vi "ELVIS-RIO Customized FPGA.vi"() -> ()   [LabVIEW 2016]
doc: "This VI contains the NI myRIO FPGA shipping personality. This VI compiles and runs on the NI myRIO FPGA target. You can modify this VI to suit your application needs. National Instruments recommends that you only add new FPGA code to this VI and do not modify the existing code. This VI might not work correctly with the myRIO VIs if you modify the existing code."
uses:
  <vilib>/Platform/TimedLoop/XDataNode/timing_clust.ctl
  <vilib>/Platform/TimedLoop/XDataNode/nitl_modes.ctl
  <vilib>/Platform/TimedLoop/XDataNode/wakeup.ctl
  <vilib>/rvi/eio/common/nirviEmuTemplateMethod_errors.vi
  <vilib>/rvi/interface/RandomDataEmulation/niFpgaRandomDataHandleErrors.vi
  <vilib>/rvi/Emulation/niFpgaCriticalErrorInLSC.vi
  <vilib>/rvi/Emulation/niFpgaGetClockAttributes.vi
  <vilib>/rvi/Emulation/niFpgaEmulationReportErrorSimple.vi
  <vilib>/rvi/Emulation/niFpgaSctlEmulationGetInTimedLoop.vi
  <vilib>/rvi/Emulation/niFpgaProcessEmulError.vi
  <vilib>/Platform/TimedLoop/XDataNode/XDataNode.xnode
  <vilib>/eio/EIONode/EIONode.xnode
  <vilib>/rvi/DataTransferAndStorage/Container/XNode/niFpgaContainer.xnode
  <vilib>/rvi/interface/RandomDataEmulation/nirviRandomDataFpgaReadWriteTemplate.vi
  <vilib>/Platform/TimedLoop/XDataNode/XDNodeRunTimeDep.lvlib
panel:
  in  "Encoder 1 Reset Value":i32
  in  "Encoder 0 Reset Value":i32
  in  "Calibrated":bool
  out "Encoder 0 Counter":i32
  out "Encoder 1 Counter":i32
  in  "Encoder 1 Reset":bool
  in  "Encoder 0 Reset":bool
  out "24V Error":bool
  in  "Camera Power":bool
  in  "LED3 Yellow":bool
  in  "LED2 Yellow":bool
  in  "LED1 Yellow":bool
  out "FIFO Receive Time Out":bool
  out "Framing Error":bool
  in  "Clear Framing Error":bool
  in  "UART Clock Divisor":u16
  in  "PWM0 Enable":bool
  out "Stall Warning 0":bool
  out "Stall Error 0":bool
  out "Encoder 0 Raw":fxp<+,2,2> format="%02b"
  out "Encoder 1 Raw":fxp<+,2,2> format="%02b"
  in  "PWM1 Enable":bool
  in  "LED1 Red":bool
  in  "LED2 Green":bool
  in  "LED2 Red":bool
  in  "LED1 Green":bool
  in  "LED3 Red":bool
  in  "LED3 Green":bool
  out "Stall Warning 1":bool
  out "Stall Error 1":bool
  out "myRIO Button":u8 format="%08b"
  in  "myRIO LED3:0":u8 format="%04b"
  in  "PWM.1A":u16
  in  "PWM.1B":u16
  in  "PWM.0A":u16
  in  "PWM.0B":u16
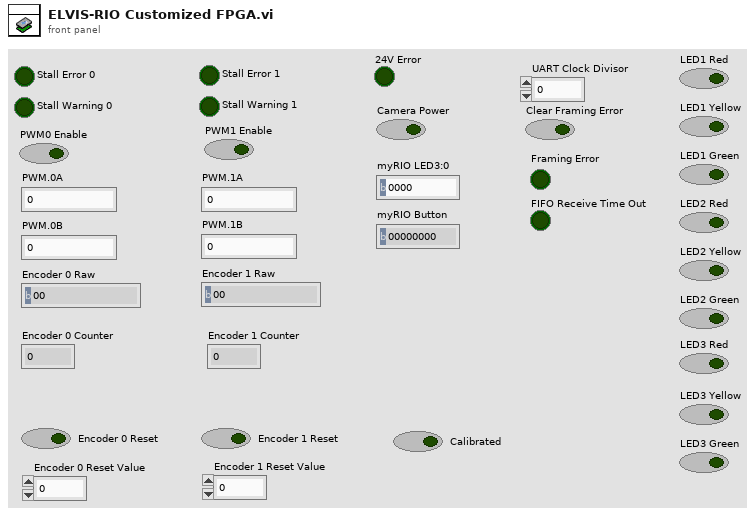
[diagram p1: front panel]
types:
  T1 = enum16{"Idle", "Testing Start", "Finish Start", "Data", "FIFO Data", "Testing Stop"}
  T2 = enum16{"Idle", "Send Bit", "Wait for Baud Period"}
  T3 = typedef "XDNodeRunTimeDep.lvlib/timing_clust.ctl" = cluster{"Expected End [f-1]":u64, "Actual End [f-1]":u64, "Finished Late? [f-1]":bool, "Expected End [i-1]":u64, "Actual End [i-1]":u64, "Finished Late? [i-1]":bool, "Expected Start [i]":u64, "Actual Start [i]":u64, "Expected Start [f]":u64, "Actual Start [f]":u64, "Source Name":string, "Structure Name":string, "Period":i64, "Deadline":i64, "Offset":i64, "Start":i64, "Priority":i32, "Timeout":i32, "Mode":T4, "Wakeup Reason":T5, "Error":errorcluster, "Source Type":string, "Secondary Source Type":string, "Global End Time":u64, "Global Start Time":u64, "Frame Duration":u64, "Iteration Duration":u64, "Assigned CPU":i32, "I/O Scan Engine Mode":u32}
  T4 = typedef "XDNodeRunTimeDep.lvlib/nitl_modes.ctl" = enum32{"No Change", "Process missed periods, maintain original phase", "Discard missed periods, maintain original phase", "Process missed periods, ignore original phase", "Discard missed periods, ignore original phase"}
  T5 = typedef "XDNodeRunTimeDep.lvlib/wakeup.ctl" = enum32{"Normal", "Aborted", "Asynchronous wakeup", "Timing source error", "Timed loop error", "Timeout"}
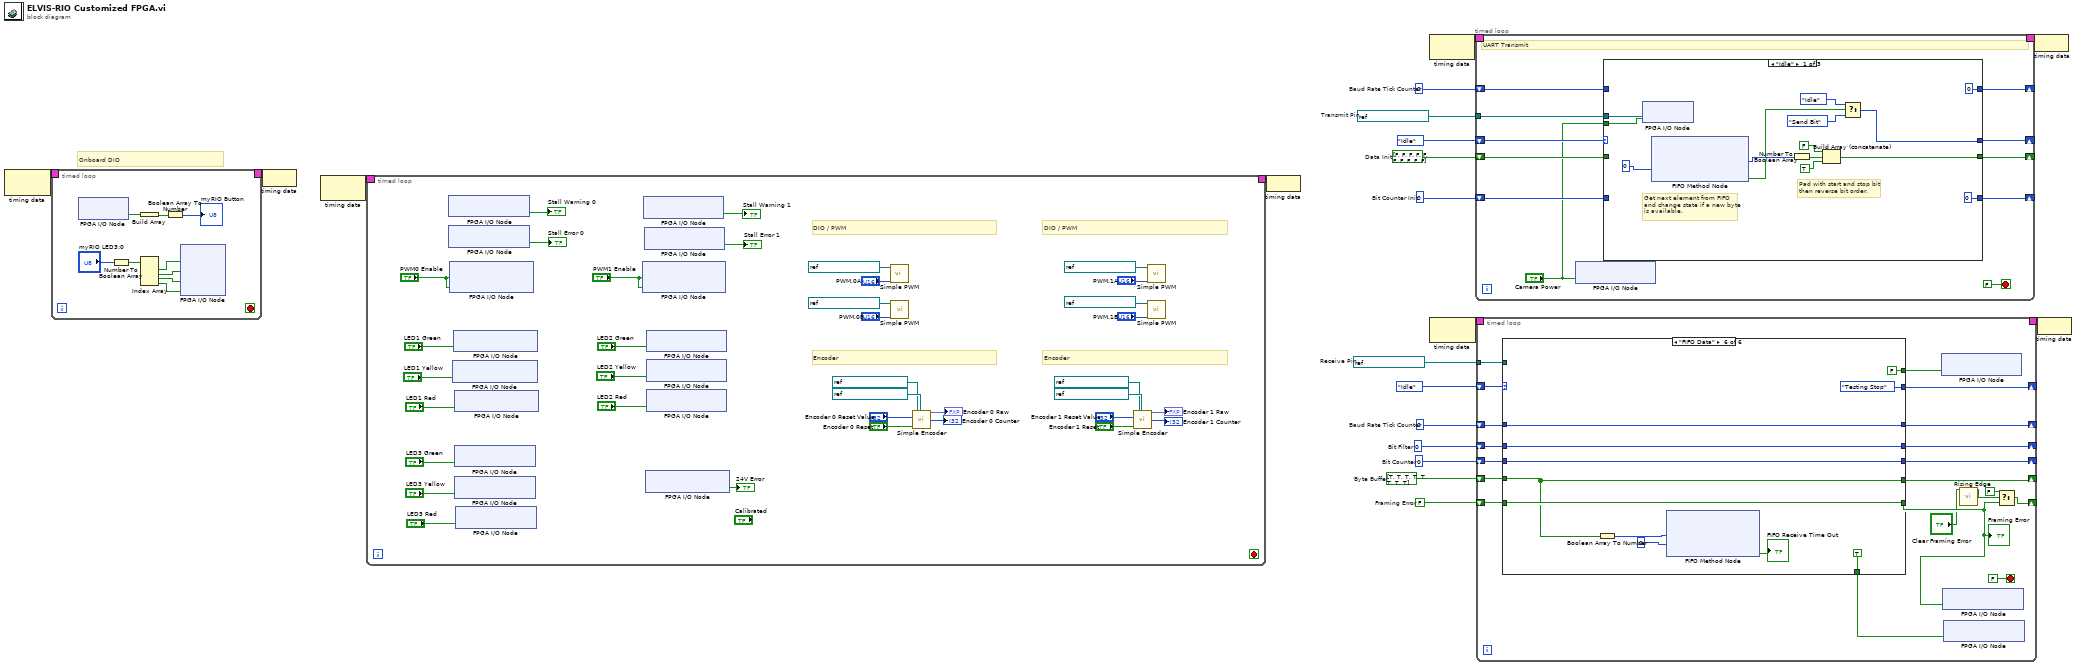
[diagram p0: block diagram]
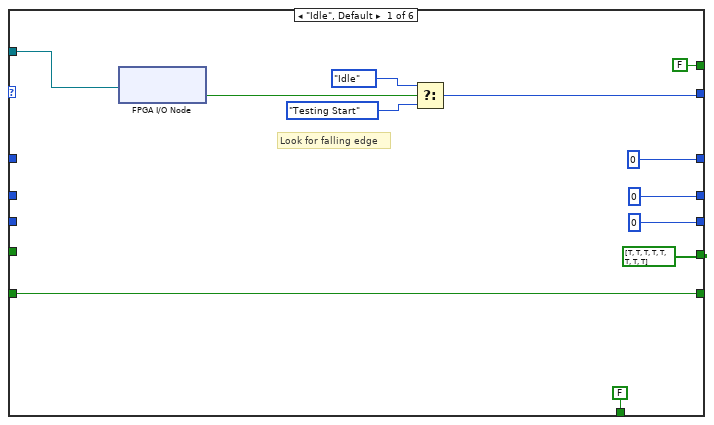
[diagram p2: hidden frame]
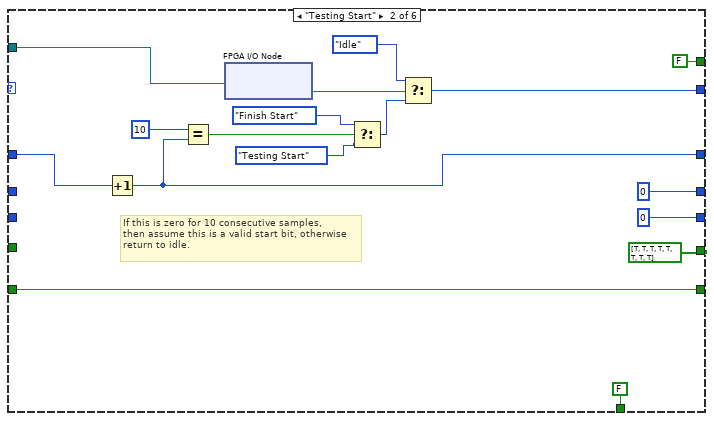
[diagram p3: hidden frame]
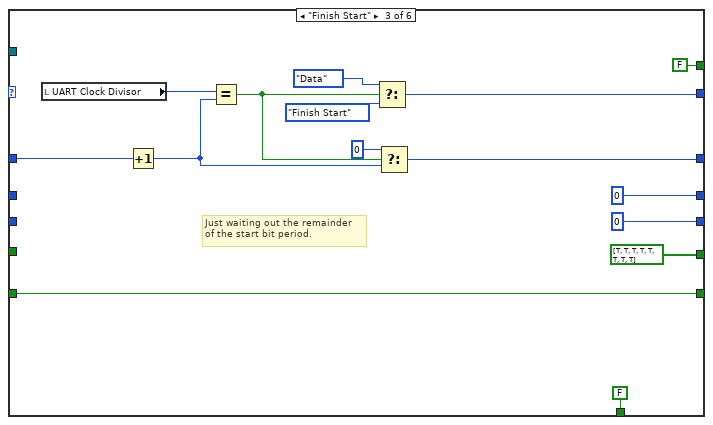
[diagram p4: hidden frame]
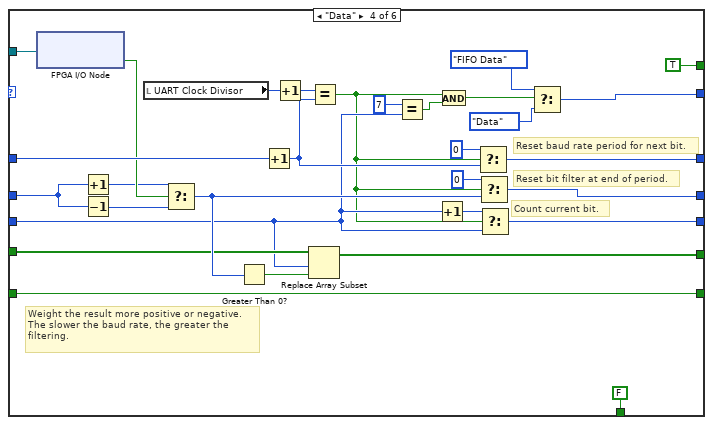
[diagram p5: hidden frame]
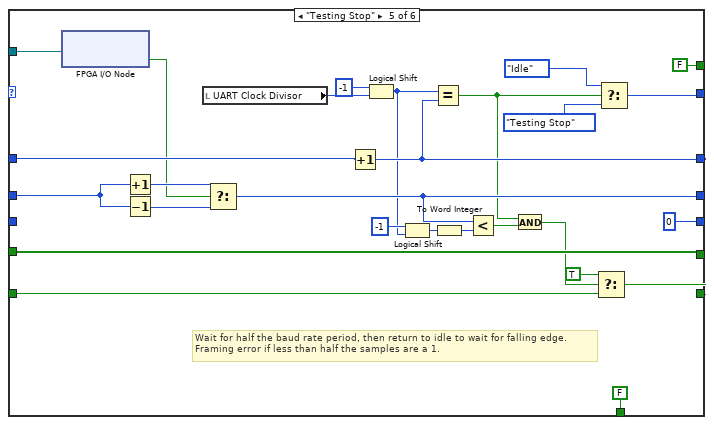
[diagram p6: hidden frame]
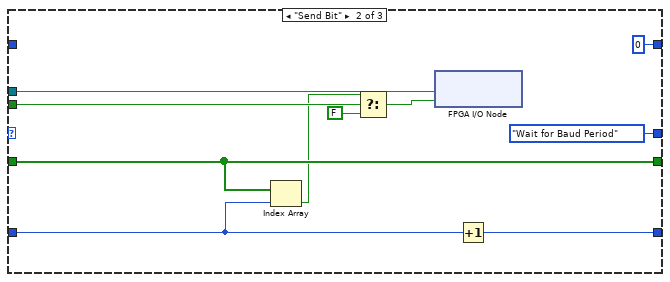
[diagram p7: hidden frame]
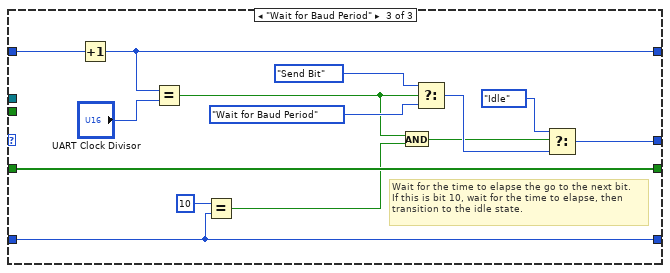
[diagram p8: hidden frame]
diagram:
  w1 = bool[] [TRUE, TRUE, TRUE, TRUE, TRUE, TRUE, TRUE, TRUE]  # Byte Buffer
  w2 = i16 0  # Bit Filter
  w3 = FALSE  # Framing Error
  w4 = u16 0  # Bit Counter
  w5 = u16 0  # Baud Rate Tick Counter
  w7 = refnum<k21> "ConnectorB/DIO3"  # Transmit Pin
  w6 = refnum<k21> "ConnectorB/DIO2"  # Receive Pin
  w9 = bool[] [FALSE, FALSE, FALSE, FALSE, FALSE, FALSE, FALSE, FALSE, FALSE, FALSE]  # Data Init
  w10 = 0  # Bit Counter Init
  w12 = u16 0  # Baud Rate Tick Counter
  # "Onboard DIO"
  n1 = node-c288() -> (w18:T3)  [unwired: 1 in]
  n2 = timed-loop {
    timing: w18 -> [_]
    timing-out: [_] -> w17
    stop <- _ stop-if-true
    n3 = xnode "FPGA I/O Node"() -> ("Button0"=w29:bool)  [unwired: 1 in, 1 out]
    n4 = Number To Boolean Array(number="myRIO LED3:0") -> (Boolean array=w25:bool[])
    n5 = Build Array(w29) -> (w28:bool[])
    n6 = Index Array(array=w25) -> (element #1=w24:bool, element #2=w23:bool, element #3=w22:bool, element #4=w21:bool)  [unwired: 4 in]
    n7 = Boolean Array To Number(Boolean array=w28) -> (number=→"myRIO Button":u8)
    n8 = xnode "FPGA I/O Node"("LED0"=w24, "LED1"=w23, "LED2"=w22, "LED3"=w21) -> ()  [unwired: 4 in, 4 out]
  }
  n9 = node-c288(w17) -> ()
  n10 = node-c288() -> (w20:T3)  [unwired: 1 in]
  n11 = timed-loop {
    timing: w20 -> [_]
    timing-out: [_] -> w19
    stop <- _ stop-if-true
    # "Encoder"
    # "DIO / PWM"
    # "Encoder"
    # "DIO / PWM"
    n12 = xnode "FPGA I/O Node"() -> ("ConnectorA/DIO0"=→"Stall Warning 0":bool)  [unwired: 1 in, 1 out]
    n13 = xnode "FPGA I/O Node"() -> ("ConnectorA/DIO1"=→"Stall Error 0":bool)  [unwired: 1 in, 1 out]
    n14 = xnode "FPGA I/O Node"("ConnectorA/DIO10"="PWM0 Enable", "ConnectorA/DIO13"="PWM0 Enable") -> ()  [unwired: 2 in, 2 out]
    n15 = xnode "FPGA I/O Node"("ConnectorA/DIO14"="LED1 Yellow") -> ()  [unwired: 1 in, 1 out]
    n16 = xnode "FPGA I/O Node"("ConnectorA/DIO15"="LED1 Green") -> ()  [unwired: 1 in, 1 out]
    n17 = xnode "FPGA I/O Node"("ConnectorA/DIO13"="LED1 Red") -> ()  [unwired: 1 in, 1 out]
    n18 = xnode "FPGA I/O Node"("ConnectorA/DIO7"="LED3 Green") -> ()  [unwired: 1 in, 1 out]
    n19 = xnode "FPGA I/O Node"("ConnectorA/DIO6"="LED3 Yellow") -> ()  [unwired: 1 in, 1 out]
    n20 = xnode "FPGA I/O Node"("ConnectorA/DIO5"="LED3 Red") -> ()  [unwired: 1 in, 1 out]
    n21 = xnode "FPGA I/O Node"("ConnectorB/DIO10"="PWM1 Enable", "ConnectorB/DIO13"="PWM1 Enable") -> ()  [unwired: 2 in, 2 out]
    n22 = xnode "FPGA I/O Node"() -> ("ConnectorB/DIO0"=→"Stall Warning 1":bool)  [unwired: 1 in, 1 out]
    n23 = xnode "FPGA I/O Node"() -> ("ConnectorB/DIO1"=→"Stall Error 1":bool)  [unwired: 1 in, 1 out]
    n24 = xnode "FPGA I/O Node"() -> ("ConnectorB/DIO15"=→"24V Error":bool)  [unwired: 1 in, 1 out]
    n25 = xnode "FPGA I/O Node"("ConnectorB/DIO6"="LED2 Yellow") -> ()  [unwired: 1 in, 1 out]
    n26 = xnode "FPGA I/O Node"("ConnectorB/DIO7"="LED2 Green") -> ()  [unwired: 1 in, 1 out]
    n27 = xnode "FPGA I/O Node"("ConnectorB/DIO5"="LED2 Red") -> ()  [unwired: 1 in, 1 out]
    n28 = call "Simple PWM.vi"("Compare Value"="PWM.0A", "PWM"=refnum<k21> "ConnectorA/DIO8" ("DIO/PWM")) -> ()  [unwired: 10 in]
    n29 = call "Simple PWM.vi"("Compare Value"="PWM.0B", "PWM"=refnum<k21> "ConnectorA/DIO9" ("DIO/PWM")) -> ()  [unwired: 10 in]
    n30 = call "Simple Encoder.vi"("Encoder Reset Value"="Encoder 0 Reset Value", "Encoder Reset"="Encoder 0 Reset", "DIO.1/QE.B"=refnum<k21> "ConnectorA/DIO11" ("DIO.0/QE.A"), "DIO.0/QE.A"=refnum<k21> "ConnectorA/DIO12" ("DIO.1/QE.B")) -> ("RAW A/B"=→"Encoder 0 Raw":fxp<+,2,2>, "Counter"=→"Encoder 0 Counter":i32)  [unwired: 14 in]
    n31 = call "Simple Encoder.vi"("Encoder Reset Value"="Encoder 1 Reset Value", "Encoder Reset"="Encoder 1 Reset", "DIO.1/QE.B"=refnum<k21> "ConnectorB/DIO11" ("DIO.0/QE.A"), "DIO.0/QE.A"=refnum<k21> "ConnectorB/DIO12" ("DIO.1/QE.B")) -> ("RAW A/B"=→"Encoder 1 Raw":fxp<+,2,2>, "Counter"=→"Encoder 1 Counter":i32)  [unwired: 14 in]
    n32 = call "Simple PWM.vi"("Compare Value"="PWM.1A", "PWM"=refnum<k21> "ConnectorB/DIO8" ("DIO/PWM")) -> ()  [unwired: 10 in]
    n33 = call "Simple PWM.vi"("Compare Value"="PWM.1B", "PWM"=refnum<k21> "ConnectorB/DIO9" ("DIO/PWM")) -> ()  [unwired: 10 in]
  }
  n34 = node-c288(w19) -> ()
  n35 = node-c288() -> (w16:T3)  [unwired: 1 in]
  n36 = node-c288() -> (w14:T3)  [unwired: 1 in]
  n37 = timed-loop {
    timing: w16 -> [_]
    timing-out: [_] -> w15
    shift-right: [w75] -> _
    shift-left: w12 -> [w76]
    shift-right: [w79] -> _
    shift-left: T2."Idle" -> [w80]
    shift-right: [w77] -> _
    shift-left: w10 -> [w78]
    shift-right: [w74] -> _
    shift-left: w9 -> [w73]
    tunnel: w7 -> [w71]
    stop <- FALSE stop-if-true
    # "UART Transmit"
    n38 = xnode "FPGA I/O Node"("ConnectorB/DIO4"="Camera Power") -> ()  [unwired: 1 in, 1 out]
    n39 = case shown="\"Idle\"" w80 {
      tunnel: [w94 T2."Wait for Baud Period" w112] -> w79
      tunnel: w78 -> [_ w104 w111]
      tunnel: [0 w103 w111] -> w77
      tunnel: w76 -> [_ _ w118]
      tunnel: [u16 0 u16 0 w117] -> w75
      tunnel: w73 -> [_ w100 w110]
      tunnel: [w86 w100 w110] -> w74
      tunnel: w71 -> [w85 w99 _]
      tunnel: "Camera Power" -> [w84 w98 _]
      frame "Idle" {
        # "Get next element from FIFO\nand change state if a new byte\nis available."
        # "Pad with start and stop bit\nthen reverse bit order."
        n40 = xnode "FPGA I/O Node"("I/O Item"=w84, "FPGA I/O In"=w85) -> ()  [unwired: 1 out]
        n41 = xnode ("FIFO Method Node")("Timeout"=0) -> ("Element"=w82:u8, "Timed Out?"=w81:bool)  [unwired: 1 in, 1 out]
        n42 = Number To Boolean Array(number=w82) -> (Boolean array=w91:bool[])
        n43 = Build Array (concatenate)(FALSE, w91, TRUE) -> (w86:bool[])
        n44 = Select(t=T2."Idle", s=w81, f=T2."Send Bit") -> (s? t:f=w94:T2)
      }
      frame "Send Bit" {
        n45 = Index Array(array=w100, index=w104) -> (element=w97:bool)
        n46 = Select(t=w97, s=w98, f=FALSE) -> (s? t:f=w96:bool)
        n47 = xnode "FPGA I/O Node"("I/O Item"=w96, "FPGA I/O In"=w99) -> ()  [unwired: 1 out]
        n48 = Increment(x=w104) -> (x+1=w103:i32)
      }
      frame "Wait for Baud Period" {
        # "Wait for the time to elapse the go to the next bit.\nIf this is bit 10, wait for the time to elapse, then \ntransition to the idle state."
        n49 = Increment(x=w118) -> (x+1=w117:u16)
        n50 = Equal?(x=w117, y="UART Clock Divisor") -> (x = y?=w106:bool)
        n51 = Equal?(x=10, y=w111) -> (x = y?=w107:bool)
        n52 = And(x=w106, y=w107) -> (x .and. y?=w105:bool)
        n53 = Select(t=T2."Send Bit", s=w106, f=T2."Wait for Baud Period") -> (s? t:f=w108:T2)
        n54 = Select(t=T2."Idle", s=w105, f=w108) -> (s? t:f=w112:T2)
      }
    }
  }
  n55 = timed-loop {
    timing: w14 -> [_]
    timing-out: [_] -> w13
    shift-right: [w126] -> _
    shift-left: T1."Idle" -> [w127]
    tunnel: w6 -> [w139]
    shift-right: [w137] -> _
    shift-left: w5 -> [w138]
    shift-right: [w136] -> _
    shift-left: w4 -> [w132]
    shift-right: [w134] -> _
    shift-left: w3 -> [w135]
    shift-right: [w130] -> _
    shift-left: w2 -> [w131]
    shift-right: [w128] -> _
    shift-left: w1 -> [w129]
    stop <- FALSE stop-if-true
    n56 = case shown="\"FIFO Data\"" w127 {
      tunnel: [w151 w167 w183 w210 w236 T1."Testing Stop"] -> w126
      tunnel: w139 -> [w150 w169 _ w202 w232 _]
      tunnel: w138 -> [_ w166 w184 w211 w241 w252]
      tunnel: [u16 0 ("Baud Rate Tick Counter") w162 w177 w209 w237 w252] -> w137
      tunnel: [u16 0 ("Baud Rate Tick Counter") u16 0 ("Baud Rate Tick Counter") u16 0 ("Baud Rate Tick Counter") w207 u16 0 ("Bit Counter") w250] -> w136
      tunnel: [w147 w160 w176 w203 w217 w249] -> w124
      tunnel: w135 -> [w147 w160 w176 w203 w219 w249]
      tunnel: w132 -> [_ _ _ w193 _ w250]
      tunnel: w131 -> [_ _ _ w200 w229 w251]
      tunnel: [i16 0 ("Bit Filter") i16 0 ("Bit Filter") i16 0 ("Bit Filter") w196 w227 w251] -> w130
      tunnel: w129 -> [_ _ _ w194 w233 w247]
      tunnel: [bool[] [TRUE, TRUE, TRUE, TRUE, TRUE, TRUE, TRUE, TRUE] ("Byte Buffer") bool[] [TRUE, TRUE, TRUE, TRUE, TRUE, TRUE, TRUE, TRUE] ("Byte Buffer") bool[] [TRUE, TRUE, TRUE, TRUE, TRUE, TRUE, TRUE, TRUE] ("Byte Buffer") w191 w233 w247] -> w128
      tunnel: [FALSE FALSE FALSE TRUE FALSE FALSE] -> w125
      tunnel: [FALSE FALSE FALSE FALSE FALSE TRUE] -> w123
      frame "Idle", Default {
        # "Look for falling edge"
        n57 = xnode "FPGA I/O Node"("FPGA I/O In"=w150) -> ("I/O Item"=w152:bool)  [unwired: 1 out]
        n58 = Select(t=T1."Idle", s=w152, f=T1."Testing Start") -> (s? t:f=w151:T1)
      }
      frame "Testing Start" {
        # "If this is zero for 10 consecutive samples,\nthen assume this is a valid start bit, otherwise\nreturn to idle."
        n59 = Increment(x=w166) -> (x+1=w162:u16)
        n60 = Equal?(x=u16 10, y=w162) -> (x = y?=w164:bool)
        n61 = xnode "FPGA I/O Node"("FPGA I/O In"=w169) -> ("I/O Item"=w168:bool)  [unwired: 1 out]
        n62 = Select(t=T1."Finish Start", s=w164, f=T1."Testing Start") -> (s? t:f=w165:T1)
        n63 = Select(t=T1."Idle", s=w168, f=w165) -> (s? t:f=w167:T1)
      }
      frame "Finish Start" {
        # "Just waiting out the remainder\nof the start bit period."
        n64 = local read "UART Clock Divisor"() -> (w182:u16)
        n65 = Increment(x=w184) -> (x+1=w180:u16)
        n66 = Equal?(x=w182, y=w180) -> (x = y?=w178:bool)
        n67 = Select(t=T1."Data", s=w178, f=T1."Finish Start") -> (s? t:f=w183:T1)
        n68 = Select(t=u16 0, s=w178, f=w180) -> (s? t:f=w177:u16)
      }
      frame "Data" {
        # "Count current bit."
        # "Reset bit filter at end of period."
        # "Reset baud rate period for next bit."
        # "Weight the result more positive or negative.\nThe slower the baud rate, the greater the\nfiltering."
        n69 = xnode "FPGA I/O Node"("FPGA I/O In"=w202) -> ("I/O Item"=w201:bool)  [unwired: 1 out]
        n70 = Increment(x=w200) -> (x+1=w198:i16)
        n71 = Decrement(x=w200) -> (x-1=w199:i16)
        n72 = local read "UART Clock Divisor"() -> (w212:u16)
        n73 = Select(t=w198, s=w201, f=w199) -> (s? t:f=w195:i16)
        n74 = Greater Than 0?(x=w195) -> (x > 0?=w192:bool)
        n75 = Increment(x=w211) -> (x+1=w213:u16)
        n76 = Increment(x=w212) -> (x+1=w187:u16)
        n77 = Replace Array Subset(array=w194, new element=w192, index=w193) -> (w191:bool[])
        n78 = Equal?(x=w187, y=w213) -> (x = y?=w188:bool)
        n79 = Equal?(x=u16 7, y=w193) -> (x = y?=w205:bool)
        n80 = Increment(x=w193) -> (x+1=w206:u16)
        n81 = And(x=w188, y=w205) -> (x .and. y?=w208:bool)
        n82 = Select(t=u16 0, s=w188, f=w213) -> (s? t:f=w209:u16)
        n83 = Select(t=i16 0, s=w188, f=w195) -> (s? t:f=w196:i16)
        n84 = Select(t=w206, s=w188, f=w193) -> (s? t:f=w207:u16)
        n85 = Select(t=T1."FIFO Data", s=w208, f=T1."Data") -> (s? t:f=w210:T1)
      }
      frame "Testing Stop" {
        # "Wait for half the baud rate period, then return to idle to wait for falling edge.\nFraming error if less than half the samples are a 1."
        n86 = xnode "FPGA I/O Node"("FPGA I/O In"=w232) -> ("I/O Item"=w228:bool)  [unwired: 1 out]
        n87 = Increment(x=w229) -> (x+1=w230:i16)
        n88 = Decrement(x=w229) -> (x-1=w231:i16)
        n89 = local read "UART Clock Divisor"() -> (w239:u16)
        n90 = Select(t=w230, s=w228, f=w231) -> (s? t:f=w227:i16)
        n91 = Increment(x=w241) -> (x+1=w237:u16)
        n92 = Logical Shift(y=i16 -1, x=w239) -> (x << y=w224:u16)
        n93 = Logical Shift(y=i16 -1, x=w224) -> (x << y=w225:u16)
        n94 = Equal?(x=w224, y=w237) -> (x = y?=w221:bool)
        n95 = To Word Integer(number=w225) -> (16bit integer=w223:i16)
        n96 = Less?(x=w227, y=w223) -> (x < y?=w222:bool)
        n97 = And(x=w221, y=w222) -> (x .and. y?=w220:bool)
        n98 = Select(t=TRUE, s=w220, f=w219) -> (s? t:f=w217:bool)
        n99 = Select(t=T1."Idle", s=w221, f=T1."Testing Stop") -> (s? t:f=w236:T1)
      }
      frame "FIFO Data" {
        n100 = Boolean Array To Number(Boolean array=w247) -> (number=w244:u8)
        n101 = xnode ("FIFO Method Node")("Element"=w244, "Timeout"=0) -> ("Timed Out?"=→"FIFO Receive Time Out":bool)  [unwired: 1 in, 1 out]
      }
    }
    "Framing Error" <- w124
    n102 = xnode "FPGA I/O Node"("ConnectorA/DIO2"=w125) -> ()  [unwired: 1 in, 1 out]
    n103 = xnode "FPGA I/O Node"("ConnectorA/DIO3"=w124) -> ()  [unwired: 1 in, 1 out]
    n104 = xnode "FPGA I/O Node"("ConnectorA/DIO4"=w123) -> ()  [unwired: 1 in, 1 out]
    n105 = call "Rising Edge.vi"("Input"="Clear Framing Error") -> ("Rise?"=w121:bool)  [unwired: 10 in]
    n106 = Select(t=FALSE, s=w121, f=w124) -> (s? t:f=w134:bool)
  }
  n107 = node-c288(w15) -> ()
  n108 = node-c288(w13) -> ()
